vi "New.vi"(11 "Entity in":refnum<class "Entity.lvclass">) -> (3 "Entity out":refnum<class "Entity.lvclass">)   [LabVIEW 2020, in "Conditu2.lvlib" / "Entity.lvclass"]
uses:
  Entity.lvclass
  Entity State.ctl
  Entity.lvclass/Entity.ctl
  Columns/ID/ID.lvclass
  Conditu2.lvlib
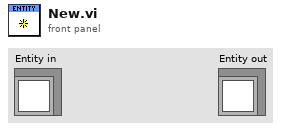
[diagram p1: front panel]
types:
  T1 = typedef "Conditu2.lvlib/Entity State.ctl" = enum16{"New", "Managed", "Detached", "Removed"}
  T2 = typedef "Conditu2.lvlib/Entity ID.ctl" = i64
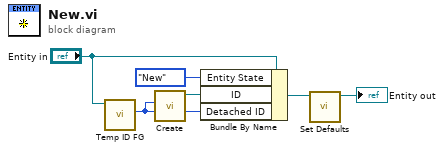
[diagram p0: block diagram]
diagram:
  n1 = call "Temp ID FG.vi"("Entity"="Entity in") -> ("New ID"=w3:T2)  [unwired: 10 in]
  n2 = call "Create.vi"("Entity ID"=w3) -> ("ID out"=w5:refnum<class "ID.lvclass">)  [unwired: 10 in]
  n3 = Bundle By Name(cluster="Entity in", "Entity State"=Entity_State."New", "ID"=w5, "Detached ID"=w3) -> (w2:refnum<class "Entity.lvclass">)
  n4 = call-dynamic "Set Defaults.vi"("Entity in"=w2) -> ("Entity out"=→"Entity out":refnum<class "Entity.lvclass">)  [unwired: 10 in]
